vi "Get All Leaves by Itemlist.vi"(8 "error in":errorcluster, 11 "Item List":T1) -> (0 "error IO":errorcluster, 3 "Children Tags":string[](array[string]))   [LabVIEW 2021]
uses:
  Control/Item List.ctl
  Control/Item Info.ctl
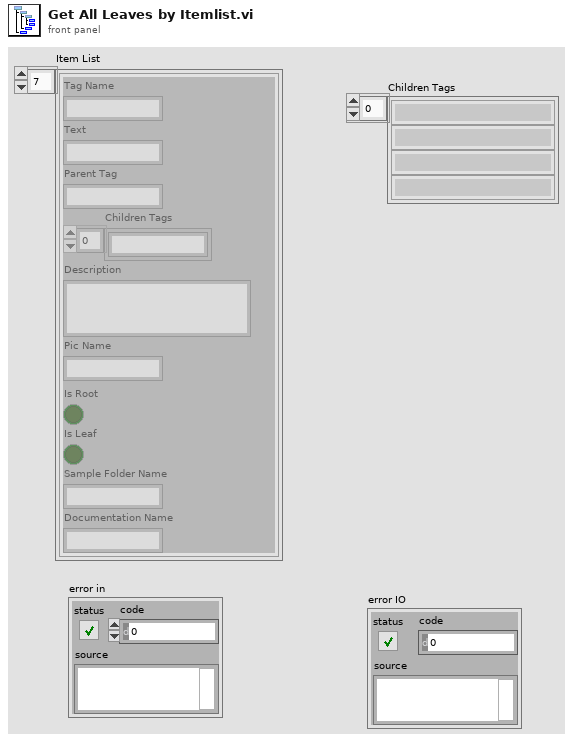
[diagram p1: front panel]
types:
  T1 = typedef "Item List.ctl" = T2[]
  T2 = typedef "Item Info.ctl" = cluster{"Tag Name":string, "Text":string, "Parent Tag":string, "Children Tags":string[], "Description":string, "Pic Name":string, "Is Root":bool, "Is Leaf":bool, "Sample Folder Name":string, "Documentation Name":string}
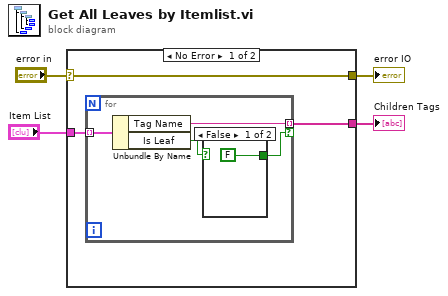
[diagram p0: block diagram]
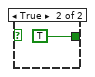
[diagram p2: hidden frame]
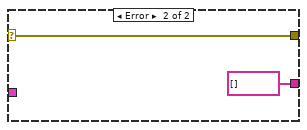
[diagram p3: hidden frame]
diagram:
  n1 = case shown="No Error" "error in" {
    selector: "error in" -> [w7 w15]
    tunnel: "Item List" -> [w6 _]
    tunnel: [w7 w15] -> w2
    tunnel: [w5 string[] []] -> w1
    frame No Error {
      n2 = for {
        tunnel: w6 -> [w10] mode=indexing
        tunnel: [w8] -> w5 mode=indexing if=w9
        n3 = Unbundle By Name(w10) -> ("Tag Name"=w8:string, "Is Leaf"=w11:bool)
        n4 = case shown="False" w11 {
          tunnel: [FALSE TRUE] -> w9
          frame False {
          }
          frame True {
          }
        }
      }
    }
    frame Error {
    }
  }
  "Children Tags" <- w1
  "error IO" <- w2
